vi "Enable.vi"(8 "error in (no error)":errorcluster, 11 "logger name":string) -> (0 "error out":errorcluster)   [LabVIEW 2018, in "GLog.lvlib" / "Registry.lvlib"]
uses:
  Registry.lvlib
  Registry Actions.ctl
panel:
  # "Connector Pane"
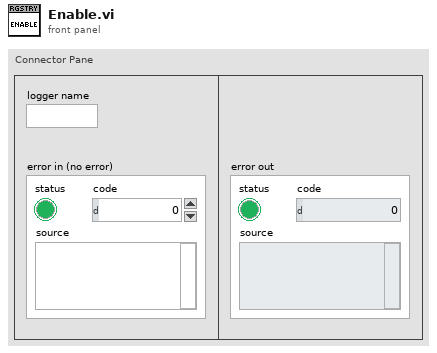
[diagram p1: front panel]
types:
  T1 = typedef "GLog.lvlib/Registry.lvlib/Registry Actions.ctl" = enum16{"Register", "Log", "Enable", "Enable All", "Disable", "Disable All", "List", "Unregister", "Unregister All"}
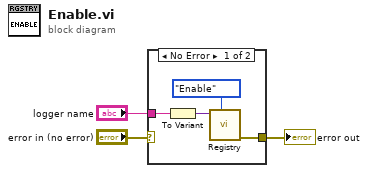
[diagram p0: block diagram]
diagram:
  n1 = case shown="No Error" "error in (no error)" {
    selector: "error in (no error)" -> [_ w8]
    tunnel: "logger name" -> [w7 _]
    tunnel: [w4 w8] -> w2
    frame No Error {
      n2 = To Variant(anything=w7) -> (Variant=w6:variant)
      n3 = call "Registry.vi"("action"=Registry_Actions."Enable", "data in"=w6) -> ("error out"=w4:errorcluster)  [unwired: 8 in, 1 out]
    }
    frame Error {
    }
  }
  "error out" <- w2
